vi "Create VO Channels.vi"(8 "error in":errorcluster, 10 "Channel Data in":T3 {"Device Chan Total" max=32 step=1; "Thermocouple"."Temperature Units" items=["Celcius", "Fahrenheit", "Kelvin", "Rankine", "Volts"]; "Thermocouple"."Thermocouple Type" items=["J", "K", "T", "E", "N", "B", "R", "S", "Raw Voltage"]}, 11 "Device Configuration Data In":T1 {"Current Section Ref" format="%.0x"; "simTC Section Refs" format="%.0x"; "Voltage Section Ref" format="%.0x"; "Custom Device Ref" format="%.0x"}) -> (0 "error out":errorcluster, 2 "Channel Data Out":T3 {"Device Chan Total" max=32 step=1; "Thermocouple"."Temperature Units" items=["Celcius", "Fahrenheit", "Kelvin", "Rankine", "Volts"]; "Thermocouple"."Thermocouple Type" items=["J", "K", "T", "E", "N", "B", "R", "S", "Raw Voltage"]}, 3 "Device Configuration Data Out":T1 {"Current Section Ref" format="%.0x"; "simTC Section Refs" format="%.0x"; "Voltage Section Ref" format="%.0x"; "Custom Device Ref" format="%.0x"})   [LabVIEW 2011, in "Simulated Thermocouple Custom Device.lvlib"]
uses:
  Simulated Thermocouple Custom Device.lvlib
  New Channel Data.ctl
  TC Selector.ctl
  TC Unit Selector.ctl
  Device Config data.ctl
  <vilib>/NI Veristand/Custom Device API/Custom Device Item Ref.ctl
  <vilib>/NI Veristand/Custom Device API/Custom Device Channel.ctl
  <vilib>/NI Veristand/Custom Device API/Custom Device Channel Type.ctl
  VO Channel Config Data.ctl
  simTC Global GUIDs.vi
  <vilib>/NI Veristand/Custom Device API/Set Item Property (Variant).vi
  <vilib>/NI Veristand/Custom Device API/Set Item Property (String).vi
  <vilib>/NI Veristand/Custom Device API/Custom Device API.lvlib
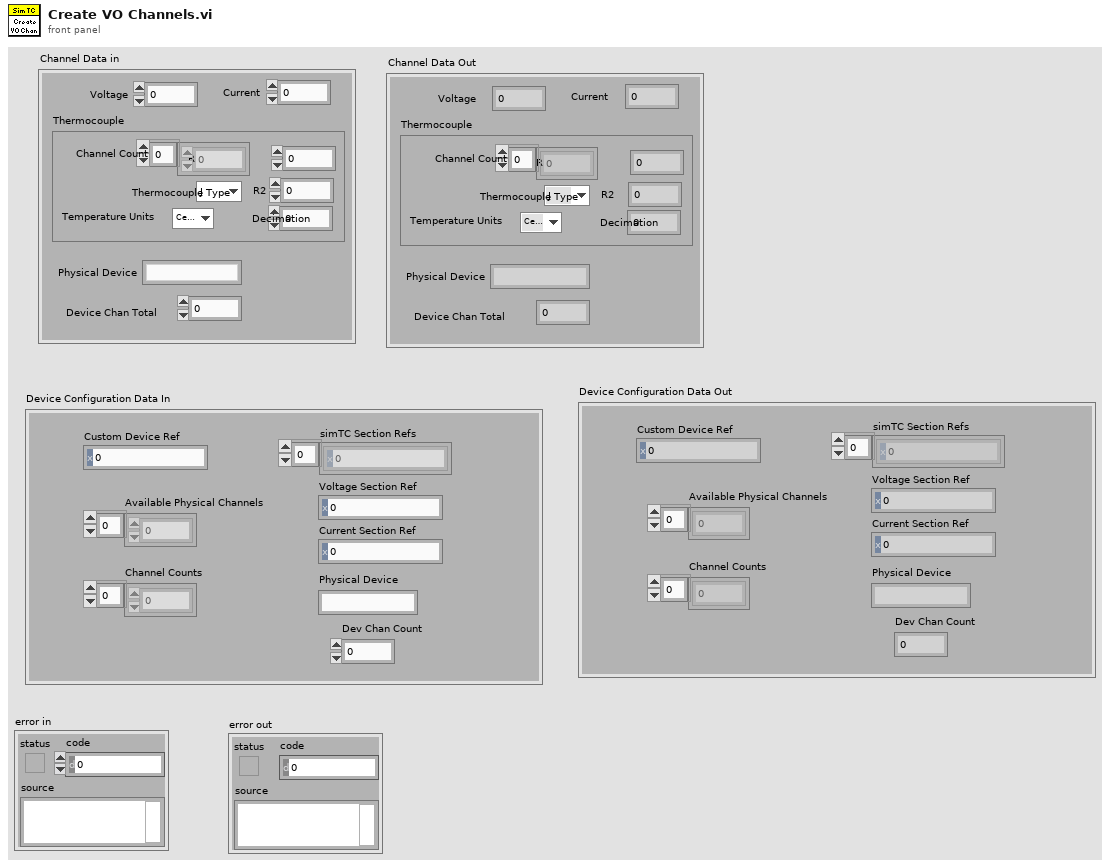
[diagram p1: front panel]
types:
  T1 = typedef "Simulated Thermocouple Custom Device.lvlib/Device Config data.ctl" = cluster{"Custom Device Ref":T2, "Voltage Section Ref":T2, "simTC Section Refs":T2[], "Current Section Ref":T2, "Physical Device":string, "Available Physical Channels":i32[], "Channel Counts":u32[], "Dev Chan Count":u32}
  T2 = typedef "Custom Device API.lvlib/Custom Device Item Ref.ctl" = u64
  T3 = typedef "Simulated Thermocouple Custom Device.lvlib/New Channel Data.ctl" = cluster{"Voltage":u32, "Current":u32, "Thermocouple":cluster{"R1":dbl, "R2":dbl, "Decimation":u32, "Thermocouple Type":T4, "Temperature Units":T5, "Channel Count":u32[]}, "Physical Device":string, "Device Chan Total":u32}
  T4 = typedef "Simulated Thermocouple Custom Device.lvlib/TC Selector.ctl" = u16
  T5 = typedef "Simulated Thermocouple Custom Device.lvlib/TC Unit Selector.ctl" = u16
  T6 = typedef "Simulated Thermocouple Custom Device.lvlib/VO Channel Config Data.ctl" = cluster{"Initial Value":dbl, "Range Min":dbl, "Range Max":dbl}
  T7 = typedef "Custom Device API.lvlib/Custom Device Channel.ctl" = cluster{"Type":T8, "Units":string, "Default Value":dbl, "Faultable":bool, "Scalable":bool}
  T8 = typedef "Custom Device API.lvlib/Custom Device Channel Type.ctl" = enum16{"Input", "Output"}
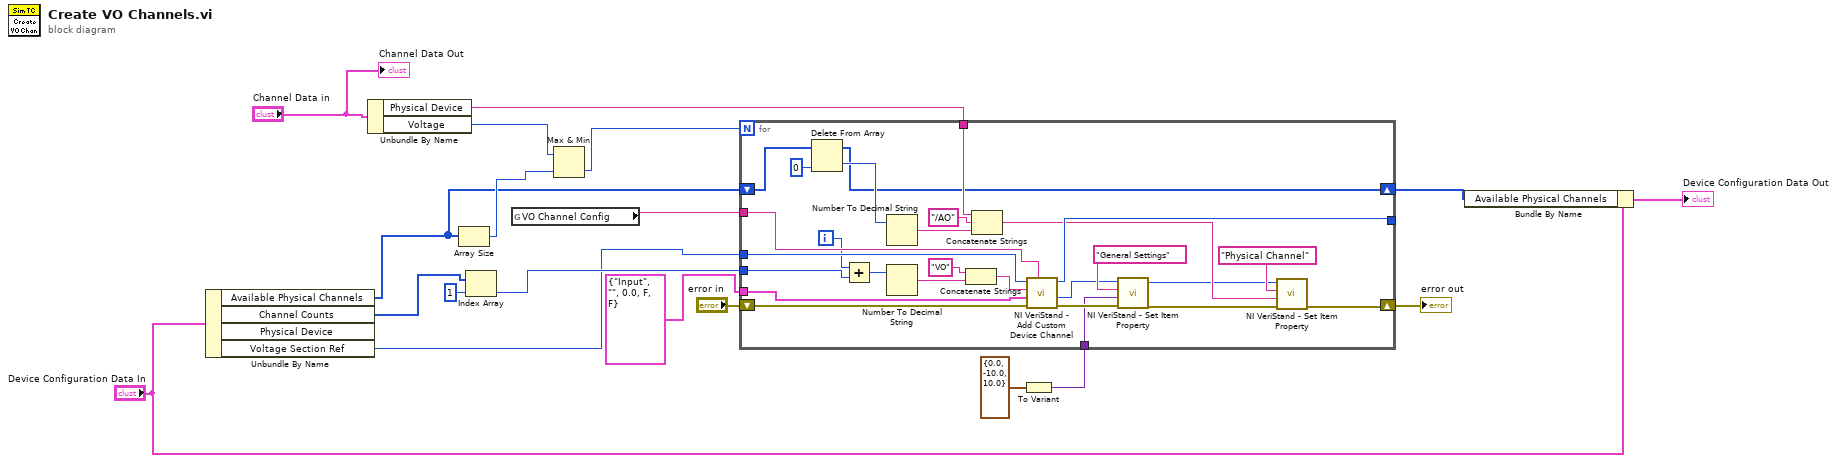
[diagram p0: block diagram]
diagram:
  n1 = Unbundle By Name("Device Configuration Data In") -> ("Available Physical Channels"=w7:i32[], "Channel Counts"=w8:u32[], "Voltage Section Ref"=w9:T2)  [unwired: 1 out]
  n2 = Unbundle By Name("Channel Data in") -> ("Physical Device"=w6:string, "Voltage"=w12:u32)
  n3 = Array Size(array=w7) -> (size(s)=w13:i32)
  n4 = Index Array(array=w8, index=1) -> (element=w15:u32)
  n5 = global read "simTC Global GUIDs.vi" "VO Channel Config"() -> (w10:string)
  n6 = Max & Min(x=w12, y=w13) -> (min(x,y)=w14:u32)  [unwired: 1 out]
  n7 = To Variant(anything=T6 {"Initial Value"=0.0, "Range Min"=-10.0, "Range Max"=10.0} ("VO Channel Config")) -> (Variant=w4:variant)
  n8 = for {
    N: w14 -> [_]
    tunnel: T7 {"Type"=enum."Input", "Units"="", "Default Value"=0.0, "Faultable"=FALSE, "Scalable"=FALSE} ("Channel") -> [w43]
    tunnel: w9 -> [w42]
    shift-right: [w24] -> w18
    shift-left: "error in" -> [w34]
    tunnel: [w41] -> _
    tunnel: w10 -> [w40]
    tunnel: w15 -> [w38]
    tunnel: w6 -> [w33]
    shift-right: [w31] -> w2
    shift-left: w7 -> [w21]
    tunnel: w4 -> [w29]
    i -> [w36]
    n9 = Delete From Array(array=w21, index=0) -> (deleted portion=w32:i32, array with subset deleted=w31:i32[])  [unwired: 1 in]
    n10 = Add(x=w36, y=w38) -> (x+y=w37:u32)
    n11 = Number To Decimal String(number=w32) -> (decimal integer string=w35:string)  [unwired: 1 in]
    n12 = Number To Decimal String(number=w37) -> (decimal integer string=w44:string)  [unwired: 1 in]
    n13 = Concatenate Strings("VO" ("Channel Name"), w44) -> (w46:string)
    n14 = Concatenate Strings(w33, "/AO", w35) -> (w25:string)
    n15 = call <vilib>:"NI VeriStand - Add Custom Device Channel.vi"("GUID (Default Channel)"=w40, "error in (no error)"=w34, "Channel"=w43, "Channel Name"=w46, "Parent Ref in"=w42) -> ("error out"=w30:errorcluster, "Channel Ref"=w23:T2, "Parent Ref out"=w41:T2)  [unwired: 3 in, 1 out]
    n16 = call-poly <vilib>:"NI VeriStand - Set Item Property.vi"("error in (no error)"=w30, "Value"=w29, "Property Name"="General Settings", "Item Ref in"=w23) -> ("error out"=w27:errorcluster, "Item Ref out"=w22:T2)  [unwired: 5 in, 1 out]
    n17 = call-poly <vilib>:"NI VeriStand - Set Item Property.vi"("error in (no error)"=w27, "Value"=w25, "Property Name"="Physical Channel", "Item Ref in"=w22) -> ("error out"=w24:errorcluster)  [unwired: 5 in, 2 out]
  }
  "error out" <- w18
  n18 = Bundle By Name(cluster="Device Configuration Data In", "Available Physical Channels"=w2) -> (→"Device Configuration Data Out":T1)
  "Channel Data Out" <- "Channel Data in"
